vi "format mapping column info.vi"(9 "instance id":string, 10 "channel":refnum<class "TBM channel.lvclass">, 11 "engine configuration in":refnum<class "engine configuration.lvclass">) -> (3 "mapping info":string)   [LabVIEW 2013, in "Table Manager.lvlib"]
uses:
  Table Manager.lvlib
  <vilib>/NI/Tag Bus Module Framework/channel/TBM channel.lvclass
  <vilib>/NI/Module Execution Interface/Engine Configuration/engine configuration.lvclass
  <vilib>/NI/Tag Bus/tag/tag descriptor.lvclass/tag descriptor.ctl
  <vilib>/NI/Tag Bus/tag/tag descriptor.lvclass
  control module/editor node/control module editor.lvclass
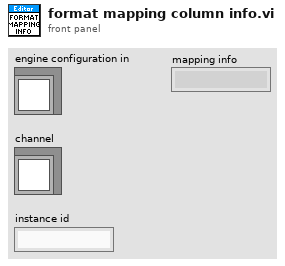
[diagram p1: front panel]
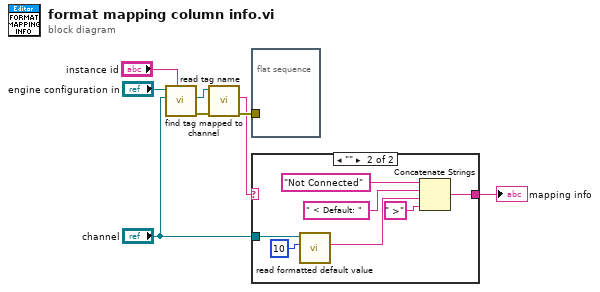
[diagram p0: block diagram]
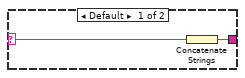
[diagram p2: hidden frame]
diagram:
  n1 = call <vilib>:"find tag mapped to channel.vi"("owner"="instance id", "channel"="channel", "engine configuration in"="engine configuration in") -> ("error out"=w5:errorcluster, "tag"=w3:refnum<class "tag descriptor.lvclass">)  [unwired: 6 in, 1 out]
  n2 = call <vilib>:"read tag name.vi"("error in"=w5, "system tag in"=w3) -> ("error out"=w8:errorcluster, "name"=w6:string)  [unwired: 7 in, 1 out]
  n3 = flat-sequence {
    tunnel: w8 -> [_]
    frame #0 {
    }
  }
  n4 = case shown="\"\"" w6 {
    selector: w6 -> [w10 _]
    tunnel: [w9 w14] -> w7
    tunnel: "channel" -> [_ w11]
    frame Default {
      n5 = Concatenate Strings(w10) -> (w9:string)
    }
    frame "" {
      n6 = call "read formatted default value.vi"("# of Digits"=10 ("y"), "channel"=w11) -> ("Formatted Default"=w12:string)  [unwired: 8 in, 1 out]
      n7 = Concatenate Strings("Not Connected", " < Default: " ("string"), w12, " >" ("string")) -> (w14:string)
    }
  }
  "mapping info" <- w7
